vi "IO@Shift__Parameter.vi"(1 "ParamterIn":string) -> (0 "ParamterOut":string)   [LabVIEW 2020]
panel:
  in  "Shift":string(combo)
  in  "PortSelect":string(combo)
  in  "Confirm":bool
  # "IO@Shift $IO1,$IO2,$IO3........(Shift=X)"
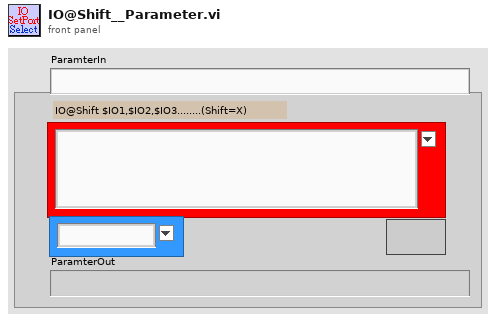
[diagram p1: front panel]
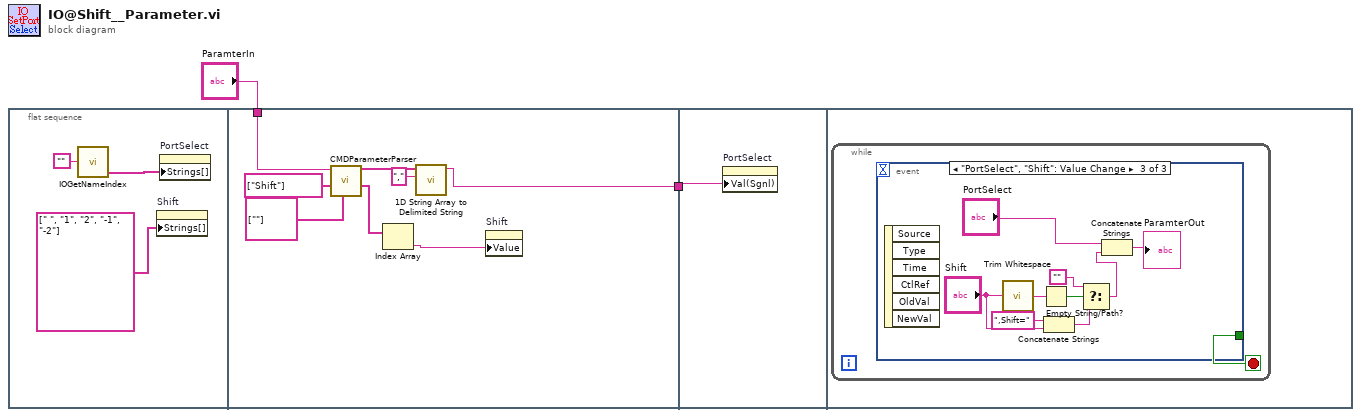
[diagram p0: block diagram]
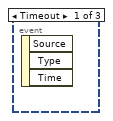
[diagram p2: hidden frame]
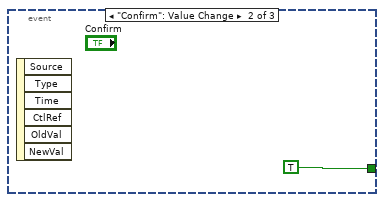
[diagram p3: hidden frame]
diagram:
  n1 = flat-sequence {
    tunnel: "ParamterIn" -> [w13]
    tunnel: [w8] -> w1
    tunnel: w1 -> [w14]
    frame #0 {
      n2 = call "IOGetNameIndex.vi"("PortName"="") -> ("PortNameList Out"=w4:string[])  [unwired: 3 in, 1 out]
      n3 = property on="Shift" class="CmbBox"("Strings[]"=string[] [" ", "1", "2", "-1", "-2"] ("Strings []")) -> ()  [unwired: 2 in, 2 out]
      n4 = property on="PortSelect" class="CmbBox"("Strings[]"=w4) -> ()  [unwired: 2 in, 2 out]
    }
    frame #1 {
      n5 = call "CMDParameterParser.vi"("DeafultValues"=string[] [""], "RequiredKeys"=string[] ["Shift"], "CMDParameter"=w13) -> ("KeyValues"=w7:string[], "Input"=w10:string[])  [unwired: 6 in, 1 out]
      n6 = Index Array(array=w7) -> (element=w6:string)  [unwired: 1 in]
      n7 = call <vilib>:"1D String Array to Delimited String.vi"("delimiter"=",", "string array"=w10) -> ("delimited string"=w8:string)  [unwired: 9 in]
      n8 = property on="Shift" class="CmbBox"("Value"=w6) -> ()  [unwired: 2 in, 2 out]
    }
    frame #2 {
      n9 = property on="PortSelect" class="CmbBox"("Val(Sgnl)"=w14) -> ()  [unwired: 2 in, 2 out]
    }
    frame #3 {
      n10 = while {
        stop <- w15 stop-if-true
        n11 = event shown="[2] \"PortSelect\", \"Shift\": Value Change" {
          selector: _ -> [_ _ _]
          dyn-events: _ -> [_ _ _]
          timeout: _ -> [_ _ _]
          tunnel: [_ TRUE _] -> w15
          event Timeout {
            n12 = event-data() -> ()  [unwired: 1 in, 3 out]
          }
          event "Confirm": Value Change {
            n13 = event-data() -> ()  [unwired: 1 in, 6 out]
          }
          event "PortSelect", "Shift": Value Change {
            n14 = event-data() -> ()  [unwired: 1 in, 6 out]
            n15 = call <vilib>:"Trim Whitespace.vi"("string"="Shift") -> ("trimmed string"=w23:string)  [unwired: 1 in]
            n16 = Empty String/Path?(string/path=w23) -> (empty?=w22:bool)
            n17 = Concatenate Strings(",Shift=" ("string"), "Shift") -> (w20:string)
            n18 = Select(t="", s=w22, f=w20) -> (s? t:f=w17:string)
            n19 = Concatenate Strings("PortSelect", w17) -> (→"ParamterOut":string)
          }
        }
      }
    }
  }
